vi "保存报警时间信息.vi"(7 "表格 5":refnum<vi>, 9 "InsertData":string[](array[string]), 11 "设备编号":i32) -> ()   [LabVIEW 2017]
uses:
  Sqlite/CBB/CreatTable.vi
  Sqlite/SQLite.lvlib
  Sqlite/CBB/InsertRowData.vi
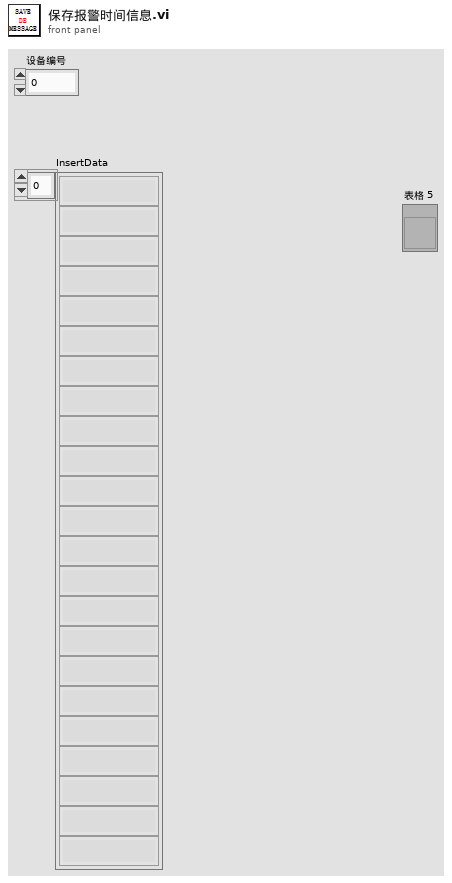
[diagram p1: front panel]
types:
  T1 = cluster{"设备明细":cluster{"table":string, "column":string[]}, "ER":cluster{"table":string, "column":string[]}}
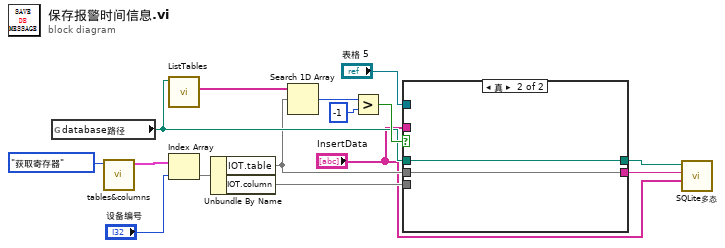
[diagram p0: block diagram]
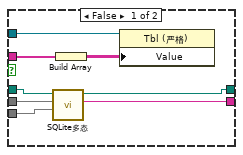
[diagram p2: hidden frame]
diagram:
  n1 = global read "全局 1.vi" "database路径"() -> (w7:path)
  n2 = call "tables&columns.vi"("选项"=enum16{"初始化", "获取寄存器"}."获取寄存器") -> ("Tables&columns"=w13:T1)  [unwired: 10 in]
  n3 = call "ListTables.vi"("DbPath"=w7) -> ("Tables"=w10:string[])  [unwired: 7 in, 3 out]
  n4 = Index Array(array=w13, index="设备编号") -> (element=w12)
  n5 = Unbundle By Name(w12) -> ("IOT.table"=w3, "IOT.column"=w5)
  n6 = Search 1D Array(1D array=w10, element=w3) -> (index of element=w9:i32)  [unwired: 1 in]
  n7 = Greater?(x=w9, y=-1) -> (0:w8:bool)
  n8 = case shown="真" w8 {
    tunnel: w7 -> [w23 w25]
    tunnel: [w22 w25] -> w6
    tunnel: w3 -> [w21 w24]
    tunnel: w5 -> [w20 _]
    tunnel: [w19 w24] -> w4
    tunnel: "表格 5" -> [w18 _]
    tunnel: "InsertData" -> [w17 _]
    frame False {
      n9 = call-poly "SQLite多态.vi"("Columns"=w20, "Table Name"=w21, "DbPath"=w23) -> ("Table Name out"=w19:string, "DbPath out"=w22:path)  [unwired: 6 in, 1 out]
      n10 = Build Array(w17) -> (w16:string[][])
      n11 = property class="Tbl (严格)"(reference=w18, "Value"=w16) -> ()  [unwired: 1 in, 2 out]
    }
    frame True {
    }
  }
  n12 = call-poly "SQLite多态.vi"("InsertData"="InsertData", "Table Name"=w4, "DbPath"=w6) -> ()  [unwired: 6 in, 3 out]
